vi "Game Engine.vi"(8 "Iteration":i32) -> (0 "Round":i32)   [LabVIEW 2015, in "SB SubVIs.lvlib"]
uses:
  SB SubVIs.lvlib
  Type Defs/Square Cluster.ctl
  Square/Square.lvclass
  Type Defs/Action Enum.ctl
  Globals.vi
  Globals (private).vi
  Type Defs/SB Type Defs.lvlib
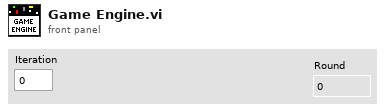
[diagram p1: front panel]
types:
  T1 = typedef "SB Type Defs.lvlib/Square Cluster.ctl" = cluster{"Attacked":bool, "Team":i32, "Next Turn":i32, "DVR":refnum<data-value>}
  T2 = typedef "SB Type Defs.lvlib/Action Enum.ctl" = enum16{"Wait", "Move", "Attack", "Replicate"}
  T3 = typedef "SB Type Defs.lvlib/Direction Enum.ctl" = enum16{"NW", "N", "NE", "E", "SE", "S", "SW", "W"}
  T4 = cluster{"Cluster":T1, i32, i32, "Action":T2, "Direction":T3, "Replicated":refnum<class "Square.lvclass">}
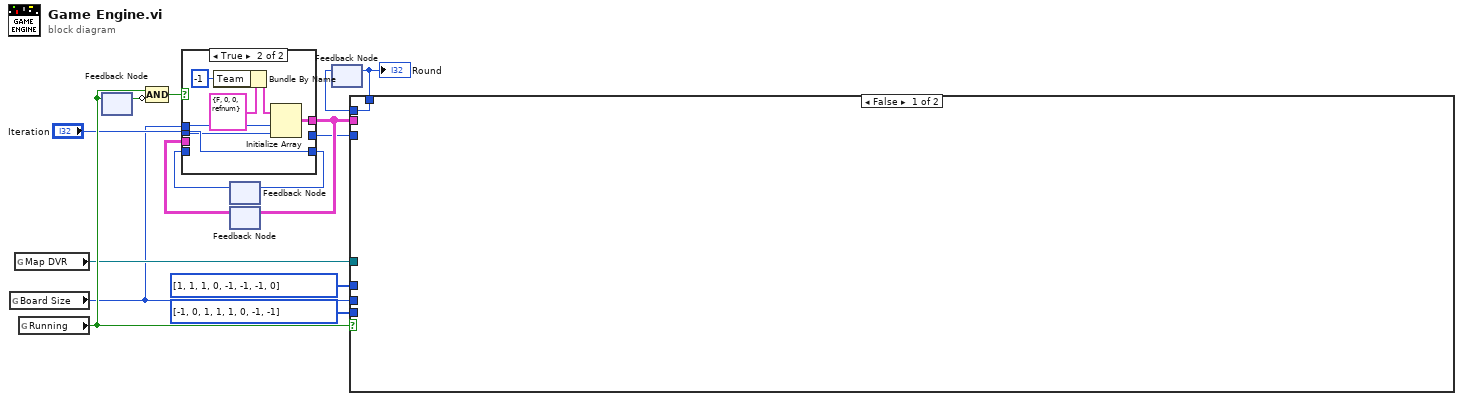
[diagram p0: block diagram]
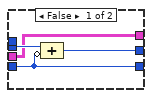
[diagram p2: hidden frame]
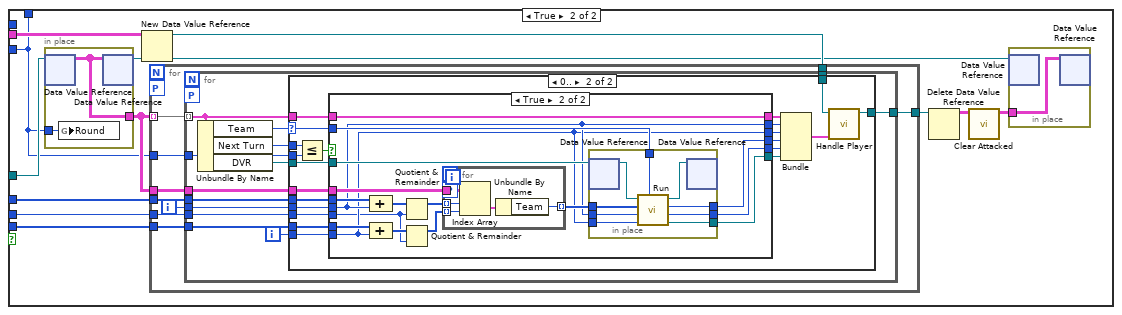
[diagram p3: hidden frame]
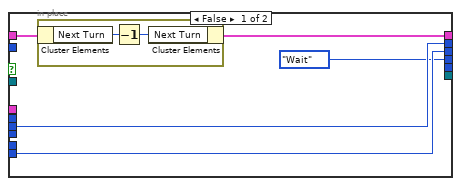
[diagram p5: hidden frame]
diagram:
  n1 = global read "Globals (private).vi" "Board Size"() -> (w3:i32)
  n2 = global read "Globals.vi" "Map DVR"() -> (w4:refnum<data-value>)
  n3 = global read "Globals.vi" "Running"() -> (w14:bool)
  n4 = feedback-in #1(w14) -> ()
  n5 = feedback #1() -> (w15:bool)  [unwired: 1 in]
  n6 = Compound Arithmetic op=AND(w14, invert w15) -> (w13:bool)
  n7 = feedback #2() -> (w10:i32)  [unwired: 1 in]
  n8 = feedback #3() -> (w9:T1[][])  [unwired: 1 in]
  n9 = case shown="True" w13 {
    tunnel: "Iteration" -> [w19 w25]
    tunnel: [w18 w25] -> w11
    tunnel: w10 -> [w18 _]
    tunnel: w3 -> [_ w24]
    tunnel: [w16 w23] -> w8
    tunnel: w9 -> [w16 _]
    tunnel: [w17 _] -> w7
    frame False {
      n10 = Compound Arithmetic op=ADD(w19, invert w18) -> (w17:i32)
    }
    frame True {
      n11 = Bundle By Name(cluster=T1 {"Attacked"=FALSE, "Team"=0, "Next Turn"=0, "DVR"=refnum} ("Cluster"), "Team"=-1) -> (w21:T1)
      n12 = Initialize Array(w21, w24, w24) -> (w23:T1[][])
    }
  }
  n13 = feedback-in #2(w11) -> ()
  n14 = feedback-in #3(w8) -> ()
  n15 = feedback #4() -> (w1:i32)  [unwired: 1 in]
  n16 = case shown="False" w14 {
    tunnel: w3 -> [_ w32]
    tunnel: w8 -> [_ w31]
    tunnel: w7 -> [_ w27]
    tunnel: i32[] [1, 1, 1, 0, -1, -1, -1, 0] -> [_ w30]
    tunnel: i32[] [-1, 0, 1, 1, 1, 0, -1, -1] -> [_ w29]
    tunnel: w4 -> [_ w28]
    tunnel: [w26 w27] -> w2
    tunnel: w1 -> [w26 _]
    frame False {
    }
    frame True {
      n17 = in-place {
        in-place-border: [w122] -> w38
        in-place-border: w27 -> [w121]
        n18 = in-place-dvr #5(w28) -> (w122:T1[][])  [unwired: 1 out]
        n19 = global write "Globals (private).vi" "Round"(w121) -> ()
        n20 = in-place-dvr #5(w122) -> (w35:refnum<data-value>)  [unwired: 1 out]
      }
      n21 = New Data Value Reference(data value=w31) -> (data value reference=w37:refnum<data-value>)  [unwired: 1 in, 1 out]
      n22 = for {
        tunnel: w38 -> [w47] mode=indexing
        tunnel: w27 -> [w46]
        tunnel: w38 -> [w45]
        tunnel: w30 -> [w44]
        tunnel: w32 -> [w42]
        tunnel: w29 -> [w41]
        tunnel: w37 -> [w40]
        tunnel: [w39] -> w36
        workers-P: _ -> [_]
        i -> [w43]
        n23 = for {
          tunnel: w47 -> [w52] mode=indexing
          tunnel: w46 -> [w51]
          tunnel: w45 -> [w60]
          tunnel: w44 -> [w59]
          tunnel: w43 -> [w58]
          tunnel: w42 -> [w57]
          tunnel: w41 -> [w56]
          workers-P: _ -> [_]
          tunnel: w40 -> [w49]
          tunnel: [w48] -> w39
          i -> [w55]
          n24 = Unbundle By Name(w52) -> ("Team"=w53:i32, "Next Turn"=w50:i32, "DVR"=w54:refnum<data-value>)
          n25 = case shown="0.." w53 {
            selector: w53 -> [_ w78]
            tunnel: w60 -> [_ w82]
            tunnel: w59 -> [_ w81]
            tunnel: w58 -> [_ w75]
            tunnel: w57 -> [_ w80]
            tunnel: w56 -> [_ w79]
            tunnel: w55 -> [_ w74]
            tunnel: w54 -> [_ w77]
            tunnel: w52 -> [_ w76]
            tunnel: w51 -> [_ w73]
            tunnel: w50 -> [_ w72]
            tunnel: w49 -> [w61 w63]
            tunnel: [w61 w62] -> w48
            frame ..-1 {
            }
            frame 0.. {
              n26 = Less Or Equal?(x=w72, y=w73) -> (x <= y?=w71:bool)
              n27 = case shown="True" w71 {
                tunnel: w82 -> [_ w106]
                tunnel: w81 -> [_ w94]
                tunnel: w80 -> [_ w90]
                tunnel: w79 -> [_ w92]
                tunnel: w78 -> [_ w99]
                tunnel: w77 -> [_ w100]
                tunnel: w76 -> [w84 w101]
                tunnel: w75 -> [w87 w93]
                tunnel: w74 -> [w86 w91]
                tunnel: [w83 w101] -> w70
                tunnel: [w87 w93] -> w69
                tunnel: [w86 w91] -> w68
                tunnel: [Action_Enum."Wait" ("Action") w105] -> w67
                tunnel: [_ w104] -> w66
                tunnel: [_ w103] -> w65
                frame False {
                  n28 = in-place {
                    n29 = in-place-cluster #6(w84) -> ("Next Turn"=w89:i32)
                    n30 = Decrement(x=w89) -> (x-1=w88:i32)
                    n31 = in-place-cluster #6("Next Turn"=w88) -> (w83:T1)
                  }
                }
                frame True {
                  n32 = Compound Arithmetic op=unknown(w94, w93) -> (w97:i32[])
                  n33 = Compound Arithmetic op=unknown(w92, w91) -> (w98:i32[])
                  n34 = Quotient & Remainder(x=w97, y=w90) -> (x-y*floor(x/y)=w96:i32[])  [unwired: 1 out]
                  n35 = Quotient & Remainder(x=w98, y=w90) -> (x-y*floor(x/y)=w95:i32[])  [unwired: 1 out]
                  n36 = for {
                    tunnel: w106 -> [w111]
                    tunnel: [w109] -> w102 mode=indexing
                    workers-P: _ -> [_]
                    tunnel: w96 -> [w108] mode=indexing
                    tunnel: w95 -> [w107] mode=indexing
                    n37 = Index Array(array=w111, index (row)=w108, index (col)=w107) -> (element=w110:T1)
                    n38 = Unbundle By Name(w110) -> ("Team"=w109:i32)
                  }
                  n39 = in-place {
                    in-place-border: [w120] -> w105
                    in-place-border: [w119] -> w104
                    in-place-border: [w118] -> w103
                    in-place-border: w102 -> [w117]
                    in-place-border: w93 -> [w116]
                    in-place-border: w91 -> [w115]
                    in-place-border: w99 -> [w112]
                    n40 = in-place-dvr #7(w100) -> (w114:refnum<class "Square.lvclass">)  [unwired: 1 out]
                    n41 = call-dynamic "Run.vi"("Team Index"=w112, "Column"=w115, "Row"=w116, "View"=w117, "Square In"=w114) -> ("Replicated"=w118:refnum<class "Square.lvclass">, "Direction"=w119:T3, "Action"=w120:T2, "Square Out"=w113:refnum<class "Square.lvclass">)  [unwired: 3 in]
                    n42 = in-place-dvr #7(w113) -> ()  [unwired: 2 out]
                  }
                }
              }
              n43 = Bundle("Cluster"=w70, w69, w68, "Action"=w67, "Direction"=w66, "Replicated"=w65) -> (w64:T4)  [unwired: 1 in]
              n44 = call "Handle Player.vi"("Move Info"=w64, "Temp DVR"=w63) -> ("Temp DVR"=w62:refnum<data-value>)  [unwired: 9 in]
            }
          }
        }
      }
      n45 = Delete Data Value Reference(data value reference=w36) -> (data value=w34:T1[][])  [unwired: 1 in, 1 out]
      n46 = call "Clear Attacked.vi"("Array in"=w34) -> ("Array out"=w33:T1[][])  [unwired: 10 in]
      n47 = in-place {
        in-place-border: w33 -> [w123]
        n48 = in-place-dvr #8(w35) -> ()  [unwired: 2 out]
        n49 = in-place-dvr #8(w123) -> ()  [unwired: 2 out]
      }
    }
  }
  "Round" <- w2
  n50 = feedback-in #4(w2) -> ()
